vi "TCP Multiple Connections - Server.vi"() -> ()   [LabVIEW 2020]
doc: "This is the TCP server VI that supports multiple connections from client VIs."
panel:
  out "Array":string[](array[string])
  in  "Stop":bool
  out "Active connections":i32
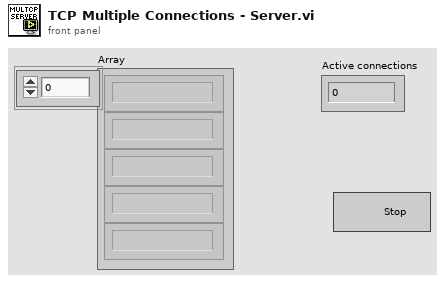
[diagram p1: front panel]
types:
  T1 = cluster{"Clients":refnum<k5>[], "Listener":refnum<k5>}
  T2 = enum16{"Initialize", "Status Check", "Send Data", "Stop", "Acquire Data"}
  T3 = enum16{"Initialize", "Status Check", "Send Data", "Stop"}
  T4 = enum16{"Standard", "Buffered", "CRLF", "Immediate"}
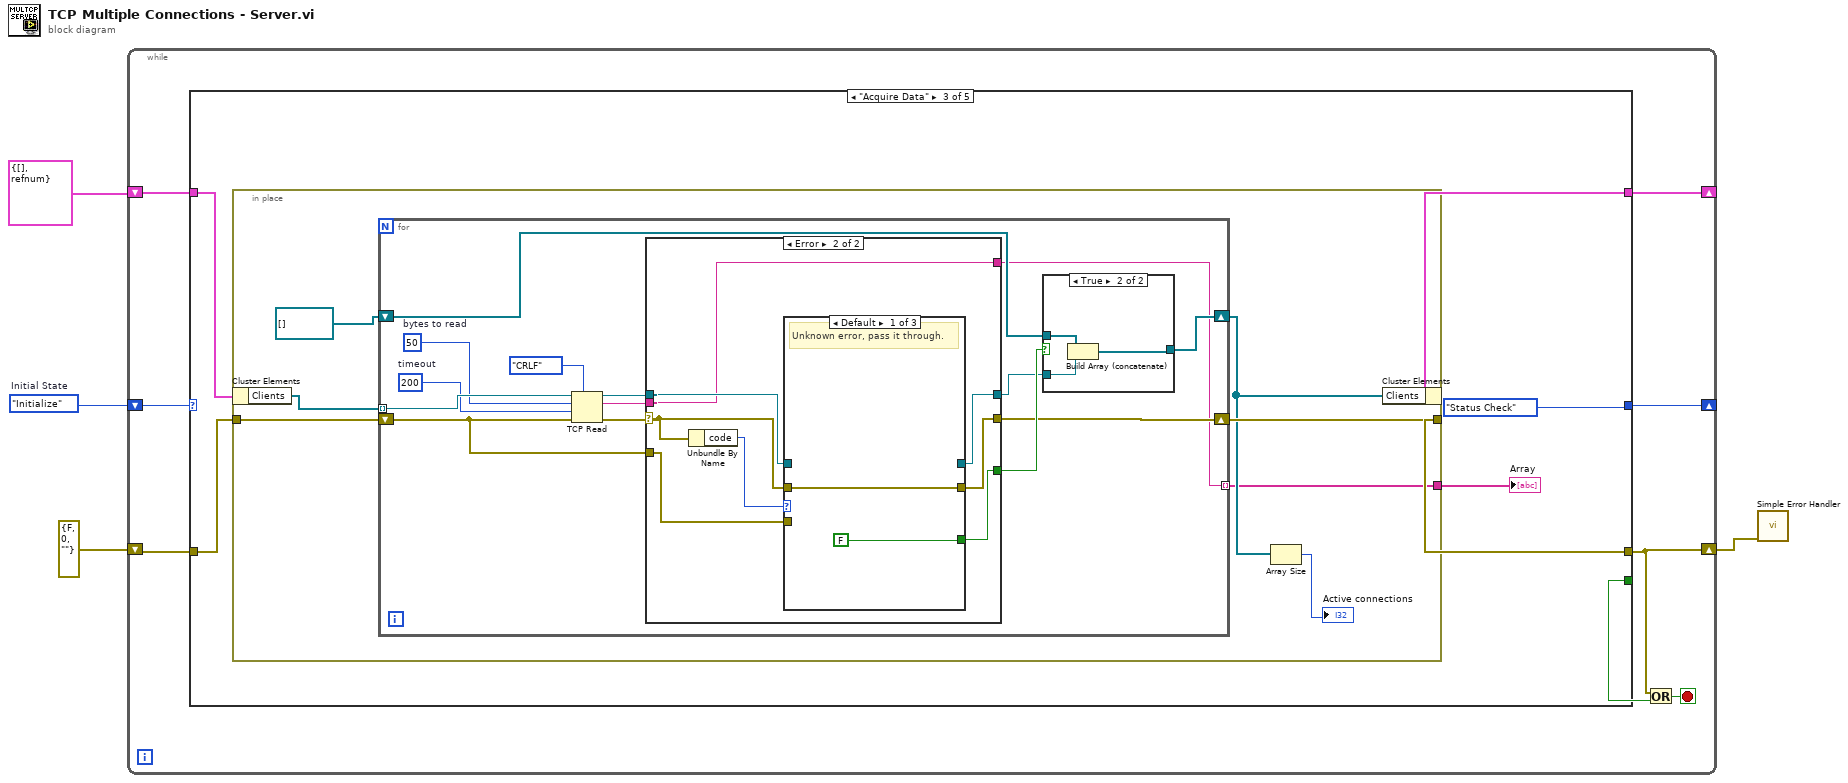
[diagram p0: block diagram]
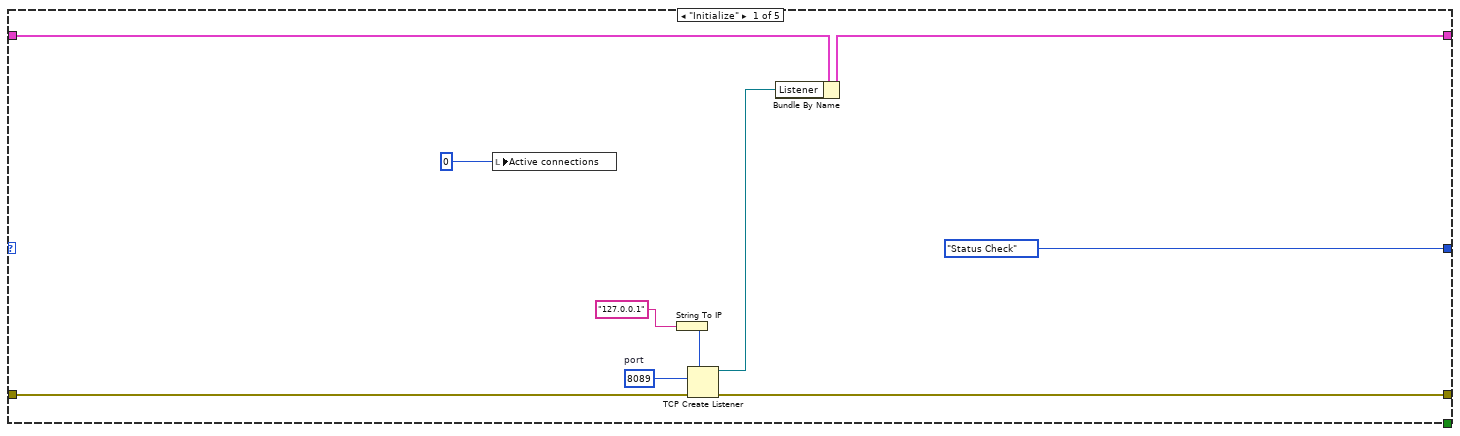
[diagram p2: hidden frame]
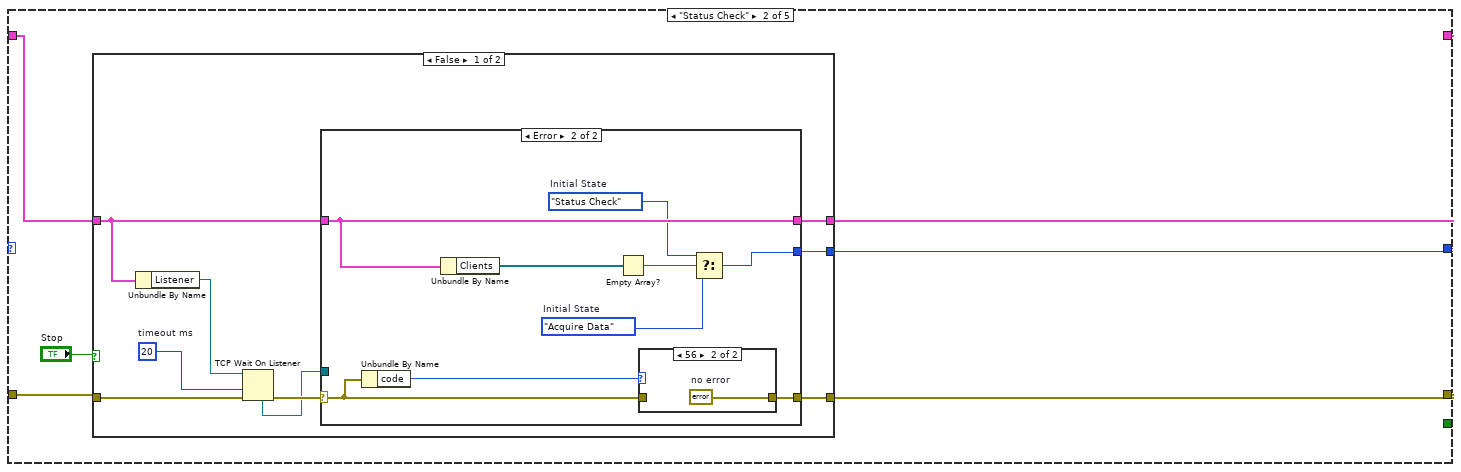
[diagram p3: hidden frame]
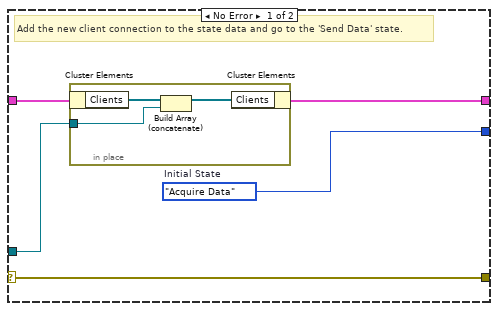
[diagram p4: hidden frame]
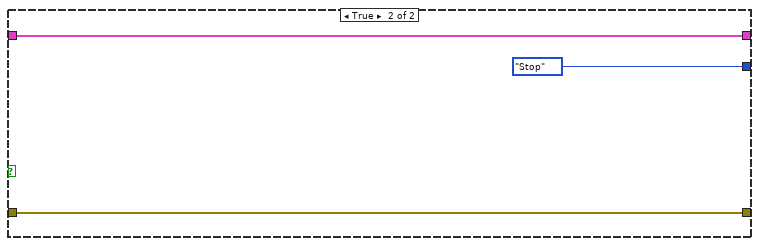
[diagram p6: hidden frame]
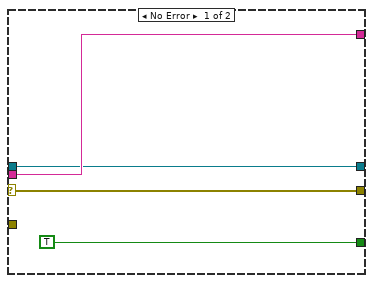
[diagram p8: hidden frame]
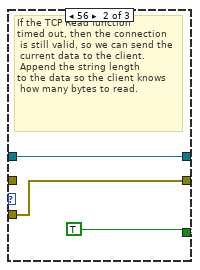
[diagram p9: hidden frame]
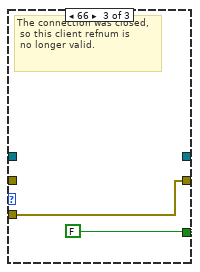
[diagram p10: hidden frame]
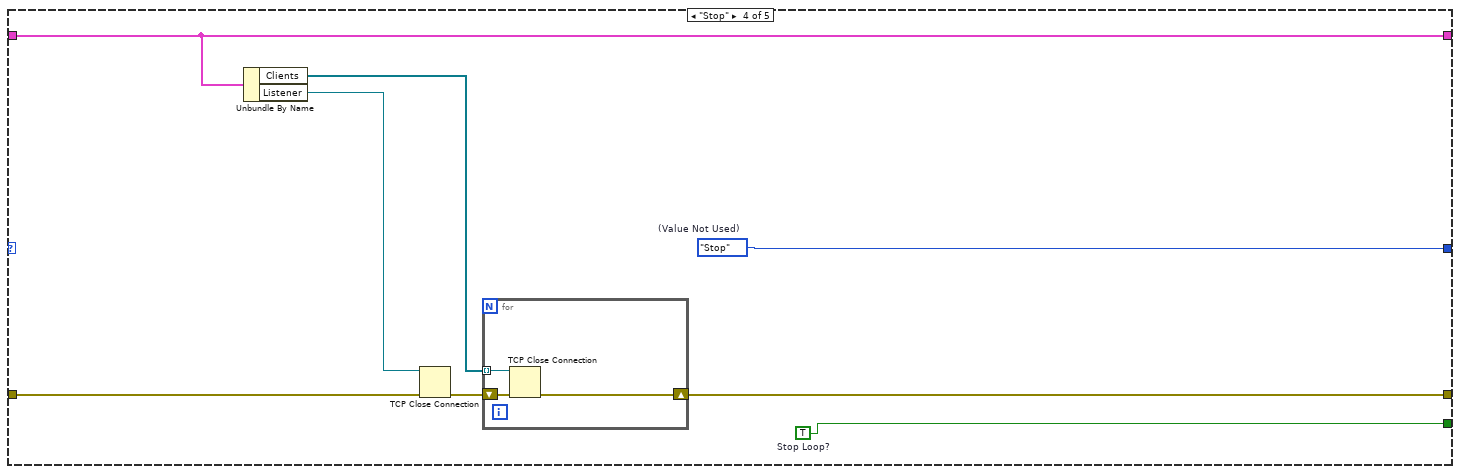
[diagram p11: hidden frame]
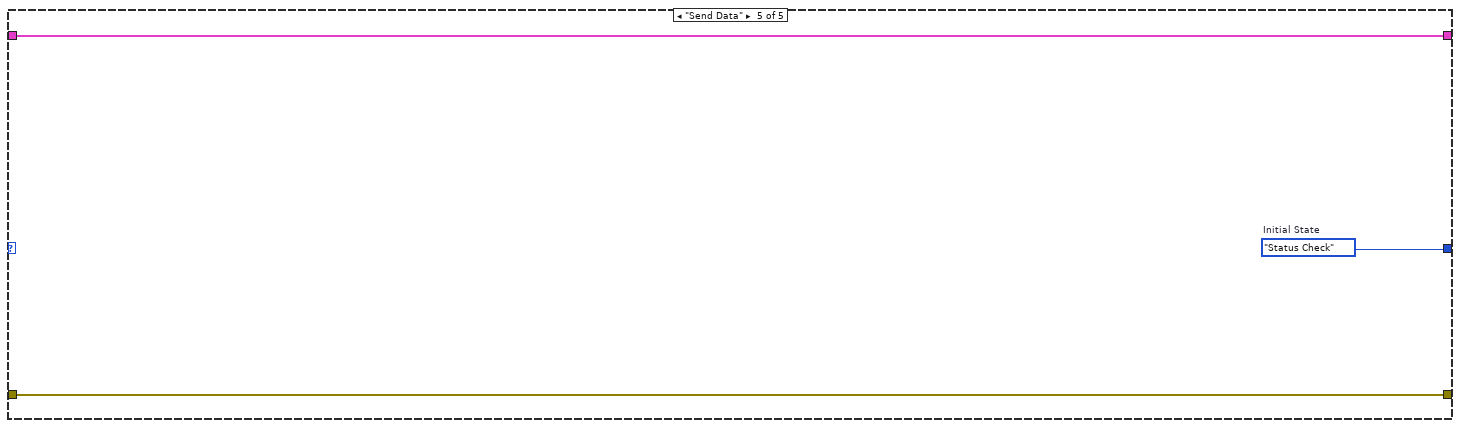
[diagram p12: hidden frame]
diagram:
  w1 = T2."Initialize"  # Initial State
  n1 = while {
    shift-right: [w11] -> _
    shift-left: w1 -> [w12]
    shift-right: [w9] -> _
    shift-left: T1 {"Clients"=[], "Listener"=refnum} ("Data") -> [w10]
    shift-right: [w5] -> w2
    shift-left: errorcluster {"status"=FALSE, "code"=0, "source"=""} ("error constant") -> [w8]
    stop <- w6 stop-if-true
    n2 = case shown="\"Acquire Data\"" w12 {
      tunnel: [T3."Status Check" ("States") w28 T3."Status Check" ("States") w110 w121] -> w11
      tunnel: [_ _ _ w117 _] -> w7
      tunnel: w10 -> [w20 w24 w63 w116 w123]
      tunnel: [w19 w23 w62 w116 w123] -> w9
      tunnel: w8 -> [w22 w27 w65 w115 w122]
      tunnel: [w21 w26 w64 w113 w122] -> w5
      frame "Initialize" {
        w17 = u16 8089  # port
        n3 = local write "Active connections"(0 ("Number of Client Connections")) -> ()
        n4 = String To IP(1:"127.0.0.1" ("service name")) -> (0:w13:u32)
        n5 = TCP Create Listener(7:w13, 8:w22, 10:w17) -> (0:w21:errorcluster, 3:w18:refnum<k5>)  [unwired: 3 out]
        n6 = Bundle By Name(cluster=w20, "Listener"=w18) -> (w19:T1)
      }
      frame "Status Check" {
        n7 = case shown="False" "Stop" {
          tunnel: [w37 T3."Stop" ("States")] -> w28
          tunnel: w27 -> [w36 w59]
          tunnel: [w29 w59] -> w26
          tunnel: w24 -> [w32 w58]
          tunnel: [w31 w58] -> w23
          frame False {
            w35 = 20  # timeout ms
            n8 = Unbundle By Name(w32) -> ("Listener"=w30:refnum<k5>)
            n9 = TCP Wait On Listener(8:w36, 9:w35, 11:w30) -> (0:w34:errorcluster, 4:w33:refnum<k5>)  [unwired: 4 out]
            n10 = case shown="Error" w34 {
              selector: w34 -> [w40 w54]
              tunnel: [w38 w48] -> w37
              tunnel: w33 -> [w41 _]
              tunnel: w32 -> [w42 w51]
              tunnel: [w39 w51] -> w31
              tunnel: [w40 w52] -> w29
              frame No Error {
                w38 = T2."Acquire Data"  # Initial State
                # "Add the new client connection to the state data and go to the 'Send Data' state."
                n11 = in-place {
                  in-place-border: w41 -> [w43]
                  n12 = in-place-cluster #1(w42) -> ("Clients"=w45:refnum<k5>[])
                  n13 = Build Array (concatenate)(w45, w43) -> (w44:refnum<k5>[])
                  n14 = in-place-cluster #1("Clients"=w44) -> (w39:T1)
                }
              }
              frame Error {
                w46 = T2."Status Check"  # Initial State
                w47 = T2."Acquire Data"  # Initial State
                n15 = Unbundle By Name(w54) -> ("code"=w53:i32)
                n16 = Unbundle By Name(w51) -> ("Clients"=w50:refnum<k5>[])
                n17 = Empty Array?(array=w50) -> (empty?=w49:bool)
                n18 = case shown="56" w53 {
                  tunnel: w54 -> [w55 _]
                  tunnel: [w55 w56] -> w52
                  frame Default {
                  }
                  frame 56 {
                    w56 = errorcluster {"status"=FALSE, "code"=0, "source"=""}  # no error
                  }
                }
                n19 = Select(t=w46, s=w49, f=w47) -> (s? t:f=w48:T2)
              }
            }
          }
          frame True {
          }
        }
      }
      frame "Acquire Data" {
        n20 = in-place {
          in-place-border: w65 -> [w72]
          in-place-border: [w71] -> w64
          in-place-border: [w66] -> w60
          n21 = in-place-cluster #2(w63) -> ("Clients"=w70:refnum<k5>[])
          n22 = for {
            tunnel: w70 -> [w86] mode=indexing
            shift-right: [w79] -> w71
            shift-left: w72 -> [w78]
            shift-right: [w76] -> w69
            shift-left: refnum<k5>[] [] ("Array") -> [w77]
            tunnel: [w73] -> w66 mode=indexing
            w83 = 200  # timeout
            w84 = 50  # bytes to read
            n23 = TCP Read(connection ID=w86, bytes to read=w84, error in (no error)=w78, 7:T4."CRLF" ("mode (standard)"), 9:w83) -> (connection ID out=w85:refnum<k5>, data out=w81:string, error out=w82:errorcluster)
            n24 = case shown="Error" w82 {
              selector: w82 -> [w93 w101]
              tunnel: w85 -> [w91 w98]
              tunnel: w81 -> [w92 w97]
              tunnel: [w91 w96] -> w75
              tunnel: [TRUE w95] -> w80
              tunnel: [w93 w100] -> w79
              tunnel: w78 -> [_ w99]
              tunnel: [w92 w97] -> w73
              frame No Error {
                # "If the client sent data, it is saying that the connection should be closed."
              }
              frame Error {
                # "Ignore connection closed and timeout errors"
                n25 = Unbundle By Name(w101) -> ("code"=w102:i32)
                n26 = case shown="Default" w102 {
                  tunnel: w101 -> [w104 _ _]
                  tunnel: [w104 w106 w109] -> w100
                  tunnel: w99 -> [_ w106 w109]
                  tunnel: w98 -> [_ w105 _]
                  tunnel: [FALSE TRUE FALSE] -> w95
                  tunnel: [_ w105 _] -> w96
                  frame Default {
                    # "Unknown error, pass it through."
                  }
                  frame 56 {
                    # "If the TCP Read function \ntimed out, then the connection\n is still valid, so we can send the\n current data to the client.\n Append the string length \nto the data so the client knows\n how many bytes to read."
                  }
                  frame 66 {
                    # "The connection was closed,\n so this client refnum is\n no longer valid."
                  }
                }
              }
            }
            n27 = case shown="True" w80 {
              tunnel: w77 -> [w87 w89]
              tunnel: w75 -> [_ w88]
              tunnel: [w87 w90] -> w76
              frame False {
              }
              frame True {
                n28 = Build Array (concatenate)(w89, w88) -> (w90:refnum<k5>[])
              }
            }
          }
          n29 = Array Size(array=w69) -> (size(s)=→"Active connections":i32)
          n30 = in-place-cluster #2("Clients"=w69) -> (w62:T1)
        }
        "Array" <- w60
      }
      frame "Stop" {
        w110 = T3."Stop"  # (Value Not Used)
        w117 = TRUE  # Stop Loop?
        n31 = Unbundle By Name(w116) -> ("Clients"=w114:refnum<k5>[], "Listener"=w111:refnum<k5>)
        n32 = TCP Close Connection(connection ID=w111, error in (no error)=w115) -> (error out=w112:errorcluster)  [unwired: 1 in, 1 out]
        n33 = for {
          shift-right: [w119] -> w113
          shift-left: w112 -> [w120]
          tunnel: w114 -> [w118] mode=indexing
          n34 = TCP Close Connection(connection ID=w118, error in (no error)=w120) -> (error out=w119:errorcluster)  [unwired: 1 in, 1 out]
        }
      }
      frame "Send Data" {
        w121 = T2."Status Check"  # Initial State
      }
    }
    n35 = Or(x=w5, y=w7) -> (x .or. y?=w6:bool)
  }
  n36 = call <vilib>:"Simple Error Handler.vi"("error in (no error)"=w2) -> ()  [unwired: 4 in, 5 out]
